vi "Msg Handler.vi"(10 "Msg":refnum<class "Msg.lvclass">, 11 "Core Actor in":refnum<class "Core Actor.lvclass">) -> (0 "Error out":errorcluster, 3 "Core Actor out":refnum<class "Core Actor.lvclass">)   [LabVIEW 2025, in "jettl.lvlib" / "Actor.lvlib" / "Core Actor.lvclass"]
uses:
  Core Actor.lvclass
  C:/git/jettl/src/jettl/jettl/Actor/Actor/Actor.lvclass
  Msg/Msg.lvclass
  Core Actor.lvclass/Core Actor.ctl
  Actor.lvlib
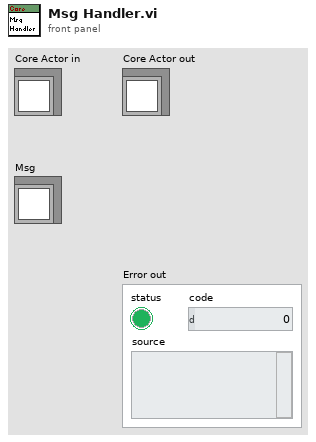
[diagram p1: front panel]
types:
  T1 = typedef "jettl.lvlib/Actor.lvlib/Msg Set.ctl" = set{refnum<class "Msg.lvclass">}
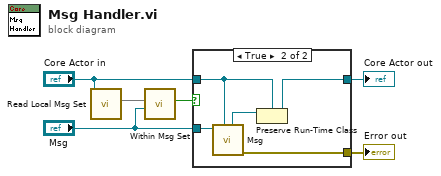
[diagram p0: block diagram]
diagram:
  n1 = call-dynamic "Read Local Msg Set.vi"("Core Actor in"="Core Actor in") -> ("Local Msg Set"=w1:T1)  [unwired: 10 in]
  n2 = call "Within Msg Set.vi"("Msg"="Msg", "Msg Set"=w1) -> ("Within Msg Set"=w6:bool)  [unwired: 9 in]
  n3 = case shown="True" w6 {
    tunnel: "Core Actor in" -> [w7 w10]
    tunnel: [w7 w9] -> w5
    tunnel: "Msg" -> [_ w12]
    tunnel: [_ w8] -> w3
    frame False {
      # "This is the inner most layer, do nothing."
    }
    frame True {
      n4 = call-dynamic "Msg.vi"("Actor in"=w10, "Msg in"=w12) -> ("Error out"=w8:errorcluster, "Actor out"=w11:refnum<class "Actor.lvclass">)  [unwired: 8 in]
      n5 = Preserve Run-Time Class(object in=w11, 2:w10) -> (object out=w9:refnum<class "Core Actor.lvclass">)  [unwired: 1 in, 1 out]
    }
  }
  "Core Actor out" <- w5
  "Error out" <- w3
